vi "EZO_sensors_tester.vi"() -> ()   [LabVIEW 2018]
panel:
  out "System Status":T1
  in  "Get Sensor Info":bool
  out "EZO Info":cluster{"ph":string, "temp":string}
  out "EZO Status":cluster{"ph":string, "temp":string}
  in  "Get Sensor Status":bool
  in  "Get Sensor Data":bool
  out "Sensor Data":cluster{"pH":sgl, "Temperature":sgl}
  out "Error Code":T2(ring)
  in  "Send Read CMD":bool
  out "Return FID":u8=2
  out "FID":u8=2
  in  "IP Address":string="192.168.5.201"
  out "System Info":T3
  out "error out":errorcluster
  in  "Get System Info":bool
  in  "Get System Status":bool
  in  "Stop":bool
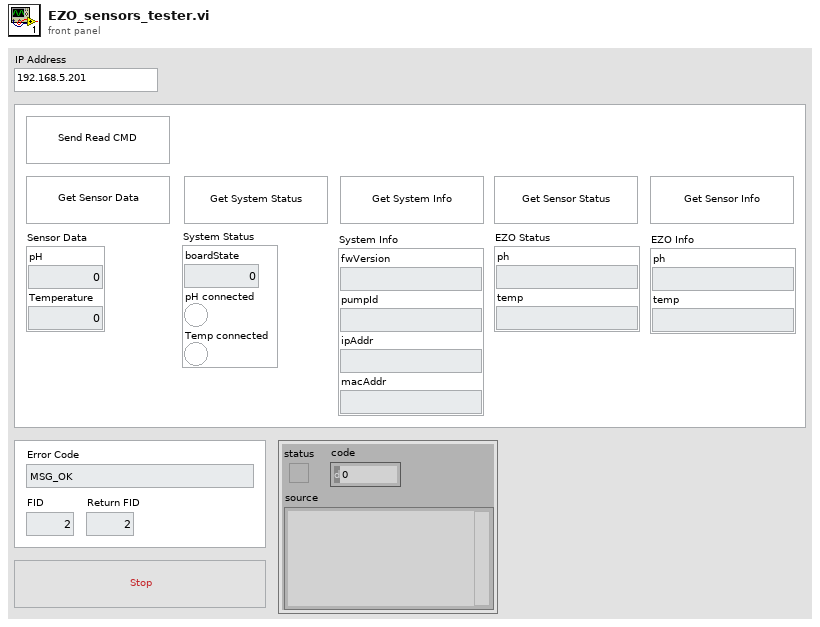
[diagram p1: front panel]
types:
  T1 = cluster{"boardState":i32, "pH connected":bool, "Temp connected":bool}
  T2 = enum16{"MSG_OK", "MSG_ERROR_NOT_SUPPORTED", "MSG_ERROR_SENSOR_DISCONNECTED", "MSG_ERROR_READING_PENDING"}
  T3 = cluster{"fwVersion":string, "pumpId":string, "ipAddr":string, "macAddr":string}
  T4 = cluster{"fwVersion":string, "pumpId":string, "macAddr":string, "ipAddr":string}
  T5 = enum16{"big-endian, network order", "native, host order", "little-endian"}
  T6 = cluster{"flowRate_mlmin":sgl, "suppliedVolume_ml":sgl}
  T7 = cluster{"pumpState":i32, "suppliedVolume_ml":sgl, "flowRate_mlmin":sgl, "home":i32, "port":i32}
  T8 = cluster{"connection ID":refnum<k5>, "header length":i32}
  T9 = cluster{"header":cluster{"length":u8, "fid":u8, "error":u8}}
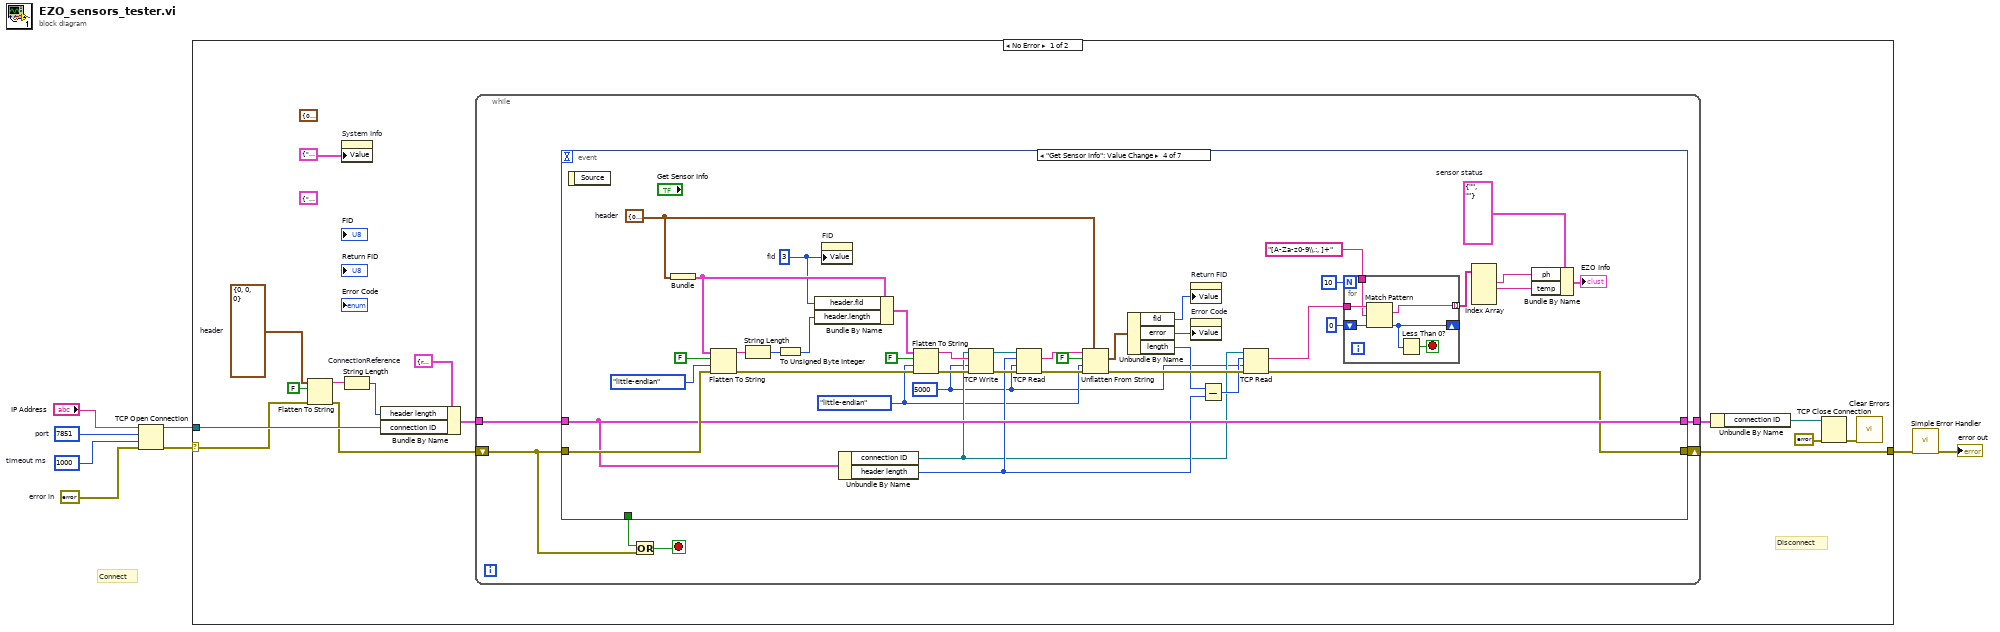
[diagram p0: block diagram]
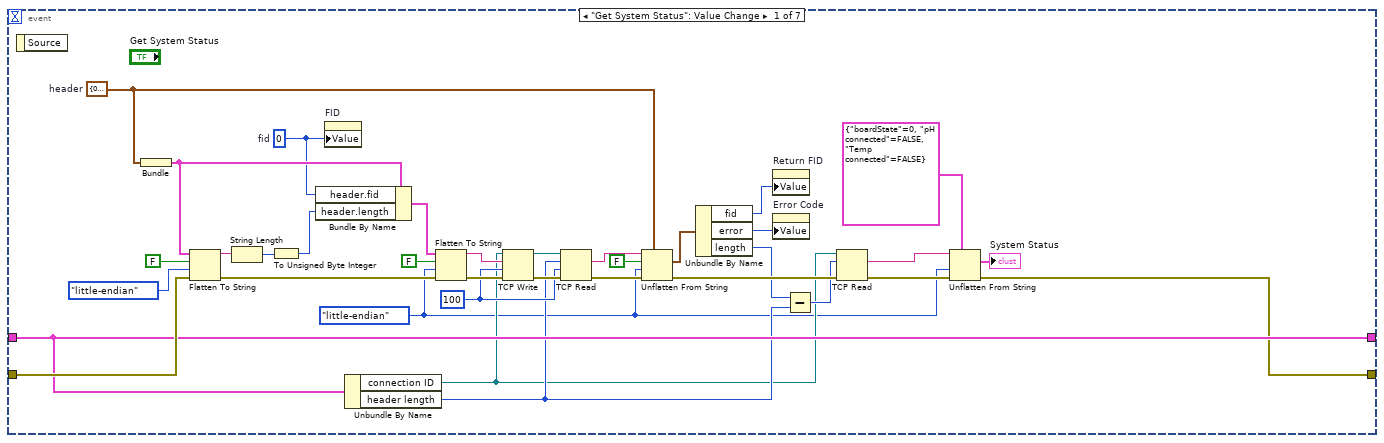
[diagram p2: hidden frame]
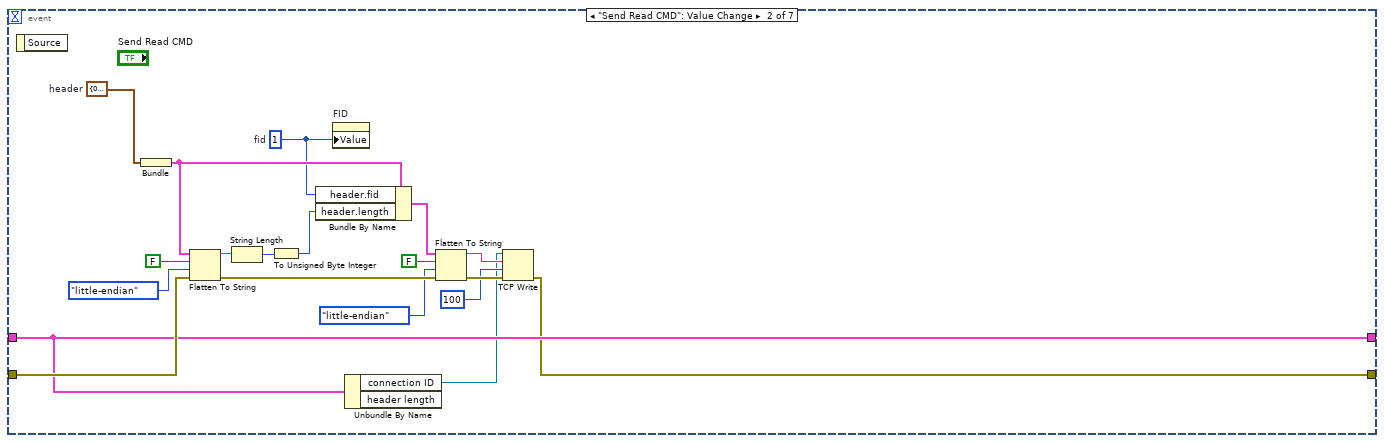
[diagram p3: hidden frame]
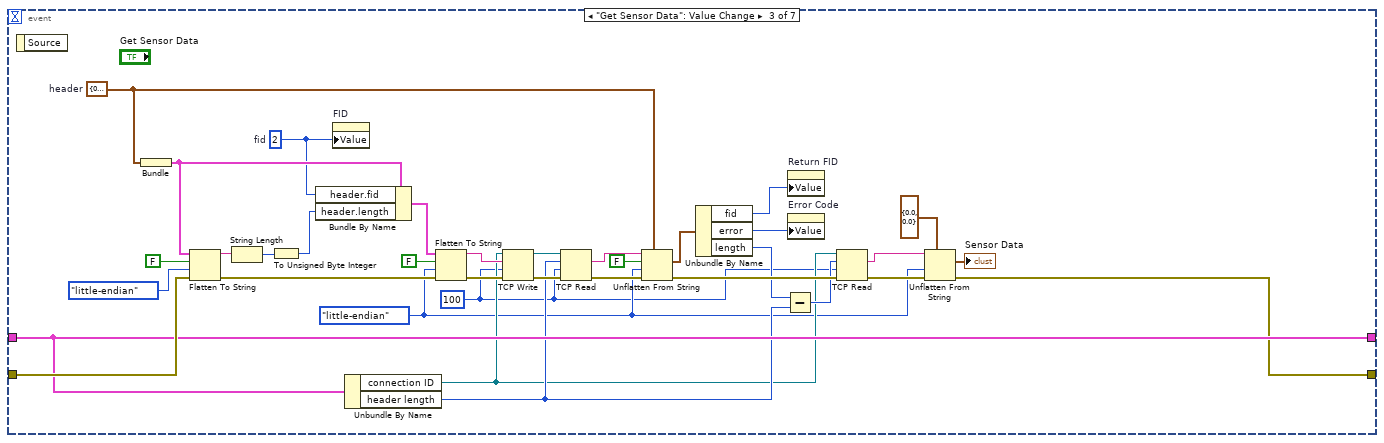
[diagram p4: hidden frame]
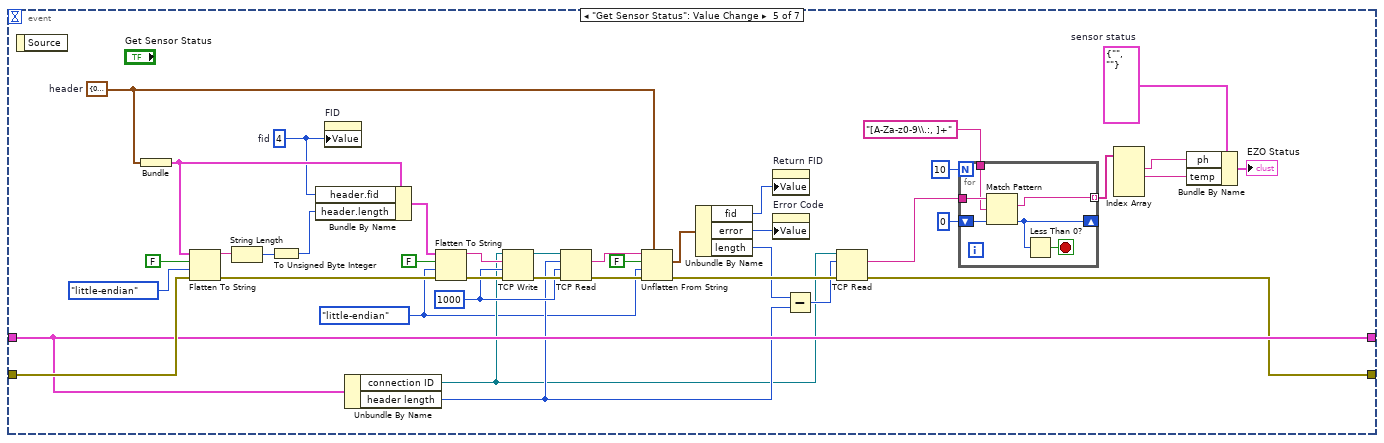
[diagram p5: hidden frame]
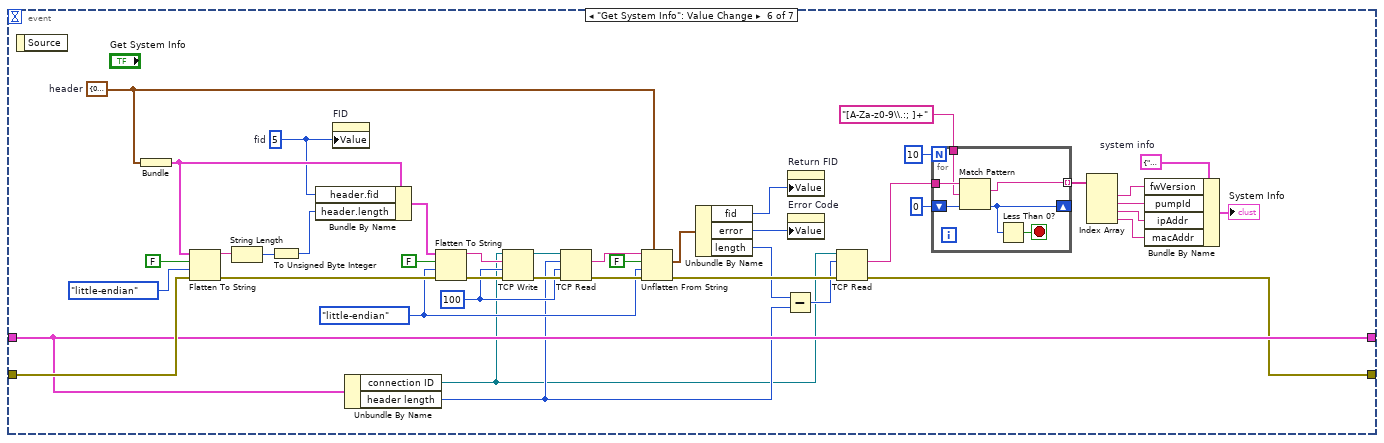
[diagram p6: hidden frame]
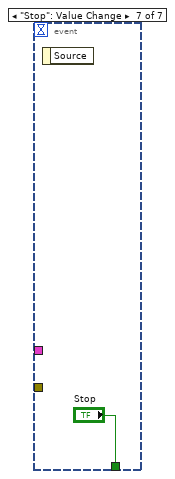
[diagram p7: hidden frame]
diagram:
  w6 = errorcluster {"status"=FALSE, "code"=0, "source"=""}  # error in
  w7 = 1000  # timeout ms
  w8 = u16 7851  # port
  # "Connect"
  n1 = TCP Open Connection(address="IP Address", remote port or service name=w8, timeout ms (60000)=w7, error in (no error)=w6) -> (connection ID=w5:refnum<k5>, error out=w1:errorcluster)  [unwired: 1 in]
  n2 = case shown="No Error" w1 {
    selector: w1 -> [w10 w260]
    tunnel: w5 -> [w19 _]
    tunnel: [w11 w260] -> w2
    frame No Error {
      (unwired) cluster{"axis":string, "stepPeriod (ms)":string} {"axis"="", "stepPeriod (ms)"=""} ("Return Motor Config")
      (unwired) T7 {"pumpState"=0, "suppliedVolume_ml"=0.0, "flowRate_mlmin"=0.0, "home"=0, "port"=0} ("Status")
      w18 = cluster{"length":u8, "fid":u8, "error":u8} {"length"=0, "fid"=0, "error"=0}  # header
      w20 = T8 {"connection ID"=refnum, "header length"=0}  # ConnectionReference
      # "Disconnect"
      n3 = Flatten To String(anything=w18, prepend array or string size? (T)=FALSE, error in (no error)=w10) -> (data string=w16:string, error out=w12:errorcluster)  [unwired: 1 in, 1 out]
      n4 = property on="System Info" class="Clust (strict)"("Value"=T4 {"fwVersion"="", "pumpId"="", "macAddr"="", "ipAddr"=""} ("system info")) -> ()  [unwired: 2 in, 2 out]
      n5 = String Length(string=w16) -> (length=w15:i32)
      n6 = Bundle By Name(cluster=w20, "header length"=w15, "connection ID"=w19) -> (w14:T8)
      n7 = while {
        tunnel: w14 -> [w29]
        tunnel: [w28] -> w13
        shift-right: [w27] -> w11
        shift-left: w12 -> [w25]
        stop <- w26 stop-if-true
        n8 = event shown="[3] \"Get Sensor Info\": Value Change" {
          selector: _ -> [_ _ _ _ _ _ _]
          dyn-events: _ -> [_ _ _ _ _ _ _]
          timeout: _ -> [_ _ _ _ _ _ _]
          tunnel: w29 -> [w53 w72 w107 w147 w193 w241 _]
          tunnel: [w53 w72 w107 w147 w193 w241 _] -> w28
          tunnel: w25 -> [w54 w73 w108 w148 w194 w242 _]
          tunnel: [w36 w65 w87 w120 w165 w218 _] -> w27
          tunnel: [_ _ _ _ _ _ "Stop"] -> w24
          event "Get System Status": Value Change {
            w45 = cluster{"length":u8, "fid":u8, "error":u8} {"length"=0, "fid"=0, "error"=0}  # header
            w47 = 100 ("timeout ms (25000)")
            w33 = u8 0  # fid
            w35 = T5."little-endian" ("byte order (0:big-endian, network order)")
            n9 = event-data() -> ()  [unwired: 1 in, 1 out]
            n10 = Bundle("header"=w45) -> (w60:T9)  [unwired: 1 in]
            n11 = Flatten To String(anything=w60, prepend array or string size? (T)=FALSE, byte order (0:big-endian, network order)=T5."little-endian", error in (no error)=w54) -> (data string=w58:string, error out=w59:errorcluster)  [unwired: 1 out]
            n12 = String Length(string=w58) -> (length=w57:i32)
            n13 = To Unsigned Byte Integer(number=w57) -> (unsigned 8bit integer=w56:u8)
            n14 = Bundle By Name(cluster=w60, "header.fid"=w33, "header.length"=w56) -> (w61:T9)
            n15 = property on="FID" class="DigNum (strict)"("Value"=w33) -> ()  [unwired: 2 in, 2 out]
            n16 = Unbundle By Name(w53) -> ("connection ID"=w39:refnum<k5>, "header length"=w41:i32)
            n17 = Flatten To String(anything=w61, prepend array or string size? (T)=FALSE, byte order (0:big-endian, network order)=w35, error in (no error)=w59) -> (data string=w63:string, error out=w64:errorcluster)  [unwired: 1 out]
            n18 = TCP Write(connection ID=w39, data in=w63, error in (no error)=w64, 9:w47) -> (connection ID out=w48:refnum<k5>, error out=w49:errorcluster)  [unwired: 1 out]
            n19 = TCP Read(connection ID=w48, bytes to read=w41, error in (no error)=w49, 9:w47) -> (data out=w50:string, error out=w51:errorcluster)  [unwired: 1 in, 1 out]
            n20 = Unflatten From String(type=w45, binary string=w50, data includes array or string size? (T)=FALSE, byte order (0:big-endian, network order)=w35, error in (no error)=w51) -> (value=w46:cluster{"length":u8, "fid":u8, "error":u8}, error out=w43:errorcluster)  [unwired: 1 out]
            n21 = Unbundle By Name(w46) -> ("fid"=w34:u8, "error"=w32:u8, "length"=w42:u8)
            n22 = property on="Return FID" class="DigNum (strict)"("Value"=w34) -> ()  [unwired: 2 in, 2 out]
            n23 = property on="Error Code" class="Enum (strict)"("Value"=w32) -> ()  [unwired: 2 in, 2 out]
            n24 = Subtract(x=w42, y=w41) -> (x-y=w40:i32)
            n25 = TCP Read(connection ID=w39, bytes to read=w40, error in (no error)=w43) -> (data out=w38:string, error out=w37:errorcluster)  [unwired: 2 in, 1 out]
            n26 = Unflatten From String(type=T1 {"boardState"=0, "pH connected"=FALSE, "Temp connected"=FALSE} ("Status"), binary string=w38, byte order (0:big-endian, network order)=w35, error in (no error)=w37) -> (value=→"System Status":T1, error out=w36:errorcluster)  [unwired: 1 in, 1 out]
          }
          event "Send Read CMD": Value Change {
            w69 = cluster{"length":u8, "fid":u8, "error":u8} {"length"=0, "fid"=0, "error"=0}  # header
            w66 = u8 1  # fid
            n27 = event-data() -> ()  [unwired: 1 in, 1 out]
            n28 = Bundle("header"=w69) -> (w79:T9)  [unwired: 1 in]
            n29 = Flatten To String(anything=w79, prepend array or string size? (T)=FALSE, byte order (0:big-endian, network order)=T5."little-endian", error in (no error)=w73) -> (data string=w77:string, error out=w78:errorcluster)  [unwired: 1 out]
            n30 = String Length(string=w77) -> (length=w76:i32)
            n31 = To Unsigned Byte Integer(number=w76) -> (unsigned 8bit integer=w75:u8)
            n32 = Bundle By Name(cluster=w79, "header.fid"=w66, "header.length"=w75) -> (w80:T9)
            n33 = property on="FID" class="DigNum (strict)"("Value"=w66) -> ()  [unwired: 2 in, 2 out]
            n34 = Unbundle By Name(w72) -> ("connection ID"=w67:refnum<k5>)  [unwired: 1 out]
            n35 = Flatten To String(anything=w80, prepend array or string size? (T)=FALSE, byte order (0:big-endian, network order)=T5."little-endian", error in (no error)=w78) -> (data string=w82:string, error out=w83:errorcluster)  [unwired: 1 out]
            n36 = TCP Write(connection ID=w67, data in=w82, error in (no error)=w83, 9:100 ("timeout ms (25000)")) -> (error out=w65:errorcluster)  [unwired: 2 out]
          }
          event "Get Sensor Data": Value Change {
            w100 = cluster{"length":u8, "fid":u8, "error":u8} {"length"=0, "fid"=0, "error"=0}  # header
            w84 = 100 ("timeout ms (25000)")
            w93 = u8 2  # fid
            w85 = T5."little-endian" ("byte order (0:big-endian, network order)")
            n37 = event-data() -> ()  [unwired: 1 in, 1 out]
            n38 = Bundle("header"=w100) -> (w114:T9)  [unwired: 1 in]
            n39 = Flatten To String(anything=w114, prepend array or string size? (T)=FALSE, byte order (0:big-endian, network order)=T5."little-endian", error in (no error)=w108) -> (data string=w112:string, error out=w113:errorcluster)  [unwired: 1 out]
            n40 = String Length(string=w112) -> (length=w111:i32)
            n41 = To Unsigned Byte Integer(number=w111) -> (unsigned 8bit integer=w110:u8)
            n42 = Bundle By Name(cluster=w114, "header.fid"=w93, "header.length"=w110) -> (w115:T9)
            n43 = property on="FID" class="DigNum (strict)"("Value"=w93) -> ()  [unwired: 2 in, 2 out]
            n44 = Unbundle By Name(w107) -> ("connection ID"=w94:refnum<k5>, "header length"=w96:i32)
            n45 = Flatten To String(anything=w115, prepend array or string size? (T)=FALSE, byte order (0:big-endian, network order)=w85, error in (no error)=w113) -> (data string=w117:string, error out=w118:errorcluster)  [unwired: 1 out]
            n46 = TCP Write(connection ID=w94, data in=w117, error in (no error)=w118, 9:w84) -> (connection ID out=w102:refnum<k5>, error out=w103:errorcluster)  [unwired: 1 out]
            n47 = TCP Read(connection ID=w102, bytes to read=w96, error in (no error)=w103, 9:w84) -> (data out=w104:string, error out=w105:errorcluster)  [unwired: 1 in, 1 out]
            n48 = Unflatten From String(type=w100, binary string=w104, data includes array or string size? (T)=FALSE, byte order (0:big-endian, network order)=w85, error in (no error)=w105) -> (value=w101:cluster{"length":u8, "fid":u8, "error":u8}, error out=w98:errorcluster)  [unwired: 1 out]
            n49 = Unbundle By Name(w101) -> ("fid"=w92:u8, "error"=w91:u8, "length"=w97:u8)
            n50 = Subtract(x=w97, y=w96) -> (x-y=w95:i32)
            n51 = property on="Return FID" class="DigNum (strict)"("Value"=w92) -> ()  [unwired: 2 in, 2 out]
            n52 = property on="Error Code" class="Enum (strict)"("Value"=w91) -> ()  [unwired: 2 in, 2 out]
            n53 = TCP Read(connection ID=w94, bytes to read=w95, error in (no error)=w98, 9:w84) -> (data out=w86:string, error out=w88:errorcluster)  [unwired: 1 in, 1 out]
            n54 = Unflatten From String(type=T6 {"flowRate_mlmin"=0.0, "suppliedVolume_ml"=0.0}, binary string=w86, byte order (0:big-endian, network order)=w85, error in (no error)=w88) -> (value=→"Sensor Data":T6, error out=w87:errorcluster)  [unwired: 1 in, 1 out]
          }
          event "Get Sensor Info": Value Change {
            w129 = cluster{"ph":string, "temp":string} {"ph"="", "temp"=""}  # sensor status
            w140 = cluster{"length":u8, "fid":u8, "error":u8} {"length"=0, "fid"=0, "error"=0}  # header
            w119 = 5000 ("timeout ms (25000)")
            w131 = u8 3  # fid
            w133 = T5."little-endian" ("byte order (0:big-endian, network order)")
            n55 = event-data() -> ()  [unwired: 1 in, 1 out]
            n56 = Bundle("header"=w140) -> (w154:T9)  [unwired: 1 in]
            n57 = Flatten To String(anything=w154, prepend array or string size? (T)=FALSE, byte order (0:big-endian, network order)=T5."little-endian", error in (no error)=w148) -> (data string=w152:string, error out=w153:errorcluster)  [unwired: 1 out]
            n58 = String Length(string=w152) -> (length=w151:i32)
            n59 = To Unsigned Byte Integer(number=w151) -> (unsigned 8bit integer=w150:u8)
            n60 = Bundle By Name(cluster=w154, "header.fid"=w131, "header.length"=w150) -> (w155:T9)
            n61 = property on="FID" class="DigNum (strict)"("Value"=w131) -> ()  [unwired: 2 in, 2 out]
            n62 = Unbundle By Name(w147) -> ("connection ID"=w134:refnum<k5>, "header length"=w136:i32)
            n63 = Flatten To String(anything=w155, prepend array or string size? (T)=FALSE, byte order (0:big-endian, network order)=w133, error in (no error)=w153) -> (data string=w157:string, error out=w158:errorcluster)  [unwired: 1 out]
            n64 = TCP Write(connection ID=w134, data in=w157, error in (no error)=w158, 9:w119) -> (connection ID out=w142:refnum<k5>, error out=w143:errorcluster)  [unwired: 1 out]
            n65 = TCP Read(connection ID=w142, bytes to read=w136, error in (no error)=w143, 9:w119) -> (data out=w144:string, error out=w145:errorcluster)  [unwired: 1 in, 1 out]
            n66 = Unflatten From String(type=w140, binary string=w144, data includes array or string size? (T)=FALSE, byte order (0:big-endian, network order)=w133, error in (no error)=w145) -> (value=w141:cluster{"length":u8, "fid":u8, "error":u8}, error out=w138:errorcluster)  [unwired: 1 out]
            n67 = Unbundle By Name(w141) -> ("fid"=w132:u8, "error"=w130:u8, "length"=w137:u8)
            n68 = property on="Return FID" class="DigNum (strict)"("Value"=w132) -> ()  [unwired: 2 in, 2 out]
            n69 = property on="Error Code" class="Enum (strict)"("Value"=w130) -> ()  [unwired: 2 in, 2 out]
            n70 = Subtract(x=w137, y=w136) -> (x-y=w135:i32)
            n71 = TCP Read(connection ID=w134, bytes to read=w135, error in (no error)=w138, 9:w119) -> (data out=w121:string, error out=w120:errorcluster)  [unwired: 1 in, 1 out]
            n72 = for {
              N: 10 -> [_]
              shift-right: [w160] -> _
              shift-left: 0 ("offset past match") -> [w164]
              tunnel: w121 -> [w163]
              tunnel: "[A-Za-z0-9\\.:, ]+" ("regular expression") -> [w162]
              tunnel: [w159] -> w125 mode=indexing
              stop <- w161 stop-if-true
              n73 = Match Pattern(string=w163, regular expression=w162, offset (0)=w164) -> (match substring=w159:string, offset past match=w160:i32)  [unwired: 2 out]
              n74 = Less Than 0?(x=w160) -> (x < 0?=w161:bool)
            }
            n75 = Index Array(array=w125) -> (element #1=w124:string, element #2=w123:string)  [unwired: 4 in, 2 out]
            n76 = Bundle By Name(cluster=w129, "ph"=w124, "temp"=w123) -> (→"EZO Info":cluster{"ph":string, "temp":string})
          }
          event "Get Sensor Status": Value Change {
            w174 = cluster{"ph":string, "temp":string} {"ph"="", "temp"=""}  # sensor status
            w185 = cluster{"length":u8, "fid":u8, "error":u8} {"length"=0, "fid"=0, "error"=0}  # header
            w187 = 1000 ("timeout ms (25000)")
            w176 = u8 4  # fid
            w178 = T5."little-endian" ("byte order (0:big-endian, network order)")
            n77 = event-data() -> ()  [unwired: 1 in, 1 out]
            n78 = Bundle("header"=w185) -> (w200:T9)  [unwired: 1 in]
            n79 = Flatten To String(anything=w200, prepend array or string size? (T)=FALSE, byte order (0:big-endian, network order)=T5."little-endian", error in (no error)=w194) -> (data string=w198:string, error out=w199:errorcluster)  [unwired: 1 out]
            n80 = String Length(string=w198) -> (length=w197:i32)
            n81 = To Unsigned Byte Integer(number=w197) -> (unsigned 8bit integer=w196:u8)
            n82 = Bundle By Name(cluster=w200, "header.fid"=w176, "header.length"=w196) -> (w201:T9)
            n83 = property on="FID" class="DigNum (strict)"("Value"=w176) -> ()  [unwired: 2 in, 2 out]
            n84 = Unbundle By Name(w193) -> ("connection ID"=w179:refnum<k5>, "header length"=w181:i32)
            n85 = Flatten To String(anything=w201, prepend array or string size? (T)=FALSE, byte order (0:big-endian, network order)=w178, error in (no error)=w199) -> (data string=w203:string, error out=w204:errorcluster)  [unwired: 1 out]
            n86 = TCP Write(connection ID=w179, data in=w203, error in (no error)=w204, 9:w187) -> (connection ID out=w188:refnum<k5>, error out=w189:errorcluster)  [unwired: 1 out]
            n87 = TCP Read(connection ID=w188, bytes to read=w181, error in (no error)=w189, 9:w187) -> (data out=w190:string, error out=w191:errorcluster)  [unwired: 1 in, 1 out]
            n88 = Unflatten From String(type=w185, binary string=w190, data includes array or string size? (T)=FALSE, byte order (0:big-endian, network order)=w178, error in (no error)=w191) -> (value=w186:cluster{"length":u8, "fid":u8, "error":u8}, error out=w183:errorcluster)  [unwired: 1 out]
            n89 = Unbundle By Name(w186) -> ("fid"=w177:u8, "error"=w175:u8, "length"=w182:u8)
            n90 = property on="Return FID" class="DigNum (strict)"("Value"=w177) -> ()  [unwired: 2 in, 2 out]
            n91 = property on="Error Code" class="Enum (strict)"("Value"=w175) -> ()  [unwired: 2 in, 2 out]
            n92 = Subtract(x=w182, y=w181) -> (x-y=w180:i32)
            n93 = TCP Read(connection ID=w179, bytes to read=w180, error in (no error)=w183) -> (data out=w166:string, error out=w165:errorcluster)  [unwired: 2 in, 1 out]
            n94 = for {
              N: 10 -> [_]
              shift-right: [w206] -> _
              shift-left: 0 ("offset past match") -> [w210]
              tunnel: w166 -> [w209]
              tunnel: "[A-Za-z0-9\\.:, ]+" ("regular expression") -> [w208]
              tunnel: [w205] -> w170 mode=indexing
              stop <- w207 stop-if-true
              n95 = Match Pattern(string=w209, regular expression=w208, offset (0)=w210) -> (match substring=w205:string, offset past match=w206:i32)  [unwired: 2 out]
              n96 = Less Than 0?(x=w206) -> (x < 0?=w207:bool)
            }
            n97 = Index Array(array=w170) -> (element #1=w169:string, element #2=w168:string)  [unwired: 4 in, 2 out]
            n98 = Bundle By Name(cluster=w174, "ph"=w169, "temp"=w168) -> (→"EZO Status":cluster{"ph":string, "temp":string})
          }
          event "Get System Info": Value Change {
            w230 = T3 {"fwVersion"="", "pumpId"="", "ipAddr"="", "macAddr"=""}  # system info
            w232 = cluster{"length":u8, "fid":u8, "error":u8} {"length"=0, "fid"=0, "error"=0}  # header
            w235 = 100 ("timeout ms (25000)")
            w213 = u8 5  # fid
            w234 = T5."little-endian" ("byte order (0:big-endian, network order)")
            n99 = event-data() -> ()  [unwired: 1 in, 1 out]
            n100 = Bundle("header"=w232) -> (w248:T9)  [unwired: 1 in]
            n101 = Flatten To String(anything=w248, prepend array or string size? (T)=FALSE, byte order (0:big-endian, network order)=T5."little-endian", error in (no error)=w242) -> (data string=w246:string, error out=w247:errorcluster)  [unwired: 1 out]
            n102 = String Length(string=w246) -> (length=w245:i32)
            n103 = To Unsigned Byte Integer(number=w245) -> (unsigned 8bit integer=w244:u8)
            n104 = Bundle By Name(cluster=w248, "header.fid"=w213, "header.length"=w244) -> (w249:T9)
            n105 = property on="FID" class="DigNum (strict)"("Value"=w213) -> ()  [unwired: 2 in, 2 out]
            n106 = Unbundle By Name(w241) -> ("connection ID"=w214:refnum<k5>, "header length"=w216:i32)
            n107 = Flatten To String(anything=w249, prepend array or string size? (T)=FALSE, byte order (0:big-endian, network order)=w234, error in (no error)=w247) -> (data string=w251:string, error out=w252:errorcluster)  [unwired: 1 out]
            n108 = TCP Write(connection ID=w214, data in=w251, error in (no error)=w252, 9:w235) -> (connection ID out=w236:refnum<k5>, error out=w237:errorcluster)  [unwired: 1 out]
            n109 = TCP Read(connection ID=w236, bytes to read=w216, error in (no error)=w237, 9:w235) -> (data out=w238:string, error out=w239:errorcluster)  [unwired: 1 in, 1 out]
            n110 = Unflatten From String(type=w232, binary string=w238, data includes array or string size? (T)=FALSE, byte order (0:big-endian, network order)=w234, error in (no error)=w239) -> (value=w233:cluster{"length":u8, "fid":u8, "error":u8}, error out=w220:errorcluster)  [unwired: 1 out]
            n111 = Unbundle By Name(w233) -> ("fid"=w212:u8, "error"=w211:u8, "length"=w217:u8)
            n112 = Subtract(x=w217, y=w216) -> (x-y=w215:i32)
            n113 = property on="Return FID" class="DigNum (strict)"("Value"=w212) -> ()  [unwired: 2 in, 2 out]
            n114 = property on="Error Code" class="Enum (strict)"("Value"=w211) -> ()  [unwired: 2 in, 2 out]
            n115 = TCP Read(connection ID=w214, bytes to read=w215, error in (no error)=w220) -> (data out=w228:string, error out=w218:errorcluster)  [unwired: 2 in, 1 out]
            n116 = for {
              N: 10 -> [_]
              shift-right: [w254] -> _
              shift-left: 0 ("offset past match") -> [w258]
              tunnel: w228 -> [w257]
              tunnel: "[A-Za-z0-9\\.:; ]+" ("regular expression") -> [w256]
              tunnel: [w253] -> w225 mode=indexing
              stop <- w255 stop-if-true
              n117 = Match Pattern(string=w257, regular expression=w256, offset (0)=w258) -> (match substring=w253:string, offset past match=w254:i32)  [unwired: 2 out]
              n118 = Less Than 0?(x=w254) -> (x < 0?=w255:bool)
            }
            n119 = Index Array(array=w225) -> (element #1=w224:string, element #2=w223:string, element #3=w222:string, element #4=w221:string)  [unwired: 4 in]
            n120 = Bundle By Name(cluster=w230, "fwVersion"=w224, "pumpId"=w223, "ipAddr"=w222, "macAddr"=w221) -> (→"System Info":T3)
          }
          event "Stop": Value Change {
            n121 = event-data() -> ()  [unwired: 1 in, 1 out]
          }
        }
        n122 = Or(x=w24, y=w25) -> (x .or. y?=w26:bool)
      }
      n123 = Unbundle By Name(w13) -> ("connection ID"=w21:refnum<k5>)
      n124 = TCP Close Connection(connection ID=w21, error in (no error)=errorcluster {"status"=FALSE, "code"=0, "source"=""}) -> (error out=w22:errorcluster)  [unwired: 1 in, 1 out]
      n125 = call <vilib>:"Clear Errors.vi"("error in (no error)"=w22) -> ()  [unwired: 5 in, 2 out]
    }
    frame Error {
    }
  }
  n126 = call <vilib>:"Simple Error Handler.vi"("error in (no error)"=w2) -> ("error out"=→"error out":errorcluster)  [unwired: 4 in, 4 out]
